vi "Close.vi"(8 "error in":errorcluster, 11 "Pressure Limit in":refnum<class "Pressure Limit.lvclass">) -> (0 "error out":errorcluster, 3 "Pressure Limit out":refnum<class "Pressure Limit.lvclass">)   [LabVIEW 2023, in "Pressure Limit.lvclass"]
uses:
  Pressure Limit.lvclass
  Pressure Limit.lvclass/Pressure Limit.ctl
  Parents/Limit/Limit.lvclass
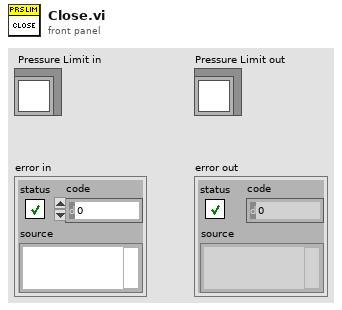
[diagram p1: front panel]
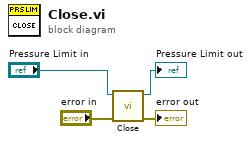
[diagram p0: block diagram]
diagram:
  n1 = call-parent "Close.vi"("error in"="error in", "Limit in"="Pressure Limit in") -> ("error out"=→"error out":errorcluster, "Limit out"=→"Pressure Limit out":refnum<class "Pressure Limit.lvclass">)  [unwired: 8 in]
